vi "OP100 Indicators.vi"(8 "error in (no error)":errorcluster, 10 "Array":refnum<vi>[](array[refnum]), 11 "OUTPUT INDICATOR in":T1) -> (0 "error out":errorcluster, 3 "OUTPUT INDICATOR out":T1)   [LabVIEW 2017]
uses:
  2f4ed2d2-b3e5-497f-b08f-b9010f661fe3.vi
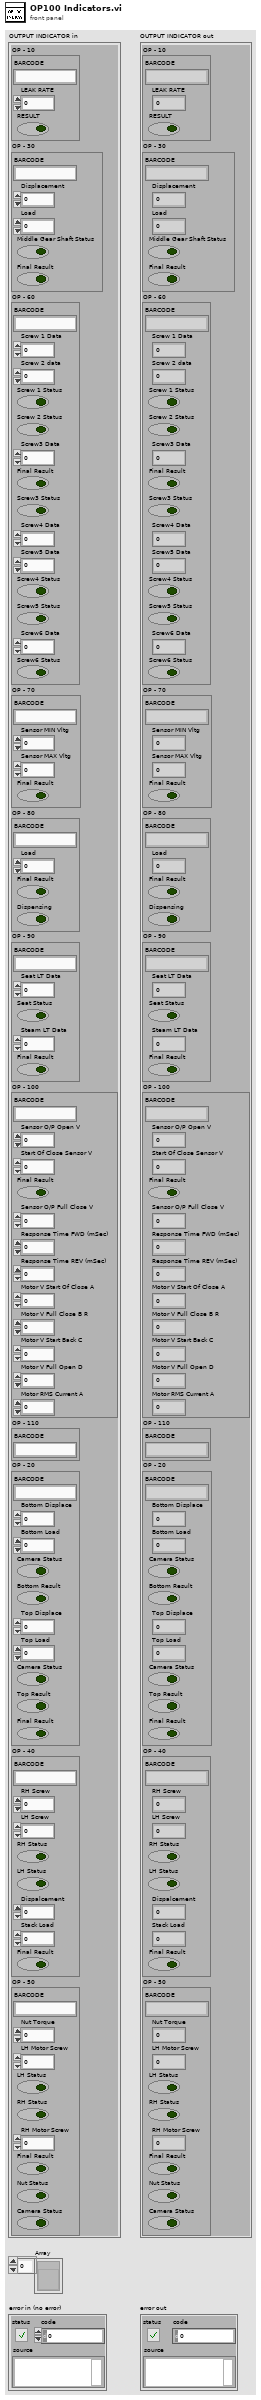
[diagram p1: front panel]
types:
  T1 = cluster{"OP - 10":cluster{"BARCODE":string, "LEAK RATE":dbl, "RESULT":bool}, "OP - 30":cluster{"BARCODE":string, "Displacement":dbl, "Load":dbl, "Middle Gear Shaft Status":bool, "Final Result":bool}, "OP - 60":cluster{"BARCODE":string, "Screw 1 Data":dbl, "Screw 2 data":dbl, "Screw 1 Status":bool, "Screw 2 Status":bool, "Screw3 Data":dbl, "Final Result":bool, "Screw3 Status":bool, "Screw4 Data":dbl, "Screw5 Data":dbl, "Screw4 Status":bool, "Screw5 Status":bool, "Screw6 Data":dbl, "Screw6 Status":bool}, "OP - 70":cluster{"BARCODE":string, "Sensor MIN Vltg":dbl, "Sensor MAX Vltg":dbl, "Final Result":bool}, "OP - 80":cluster{"BARCODE":string, "Load":dbl, "Final Result":bool, "Dispensing":bool}, "OP - 90":cluster{"BARCODE":string, "Seat LT Data":dbl, "Seat Status":bool, "Steam LT Data":dbl, "Final Result":bool}, "OP - 100":cluster{"BARCODE":string, "Sensor O/P Open V":dbl, "Start Of Close Sensor V":dbl, "Final Result":bool, "Sensor O/P Full Close V":dbl, "Response Time FWD (mSec)":dbl, "Response Time REV (mSec)":dbl, "Motor V Start Of Close A":dbl, "Motor V Full Close B R":dbl, "Motor V Start Back C":dbl, "Motor V Full Open D":dbl, "Motor RMS Current A":dbl}, "OP - 110":cluster{"BARCODE":string}, "OP - 20":cluster{"BARCODE":string, "Bottom Displace":dbl, "Bottom Load":dbl, "Camera Status":bool, "Bottom Result":bool, "Top Displace":dbl, "Top Load ":dbl, "Camera Status":bool, "Top Result":bool, "Final Result":bool}, "OP - 40":cluster{"BARCODE":string, "RH Screw":dbl, "LH Screw ":dbl, "RH Status":bool, "LH Status":bool, "Dispalcement ":dbl, "Stack Load ":dbl, "Final Result":bool}, "OP - 50":cluster{"BARCODE":string, "Nut Torque":dbl, "LH Motor Screw":dbl, "LH Status":bool, "RH Status":bool, "RH Motor Screw":dbl, "Final Result":bool, "Nut Status":bool, "Camera Status":bool}}
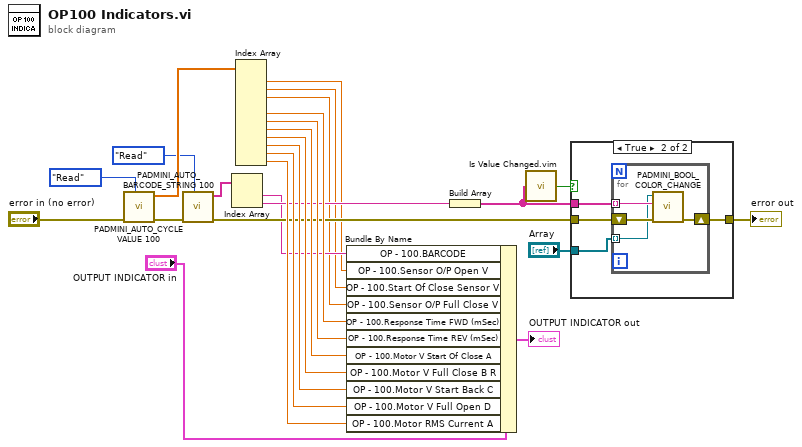
[diagram p0: block diagram]
diagram:
  n1 = call "PADMINI_AUTO_CYCLE VALUE 100.vi"("Enum"=enum16{"Read", "Write"}."Read", "error in (no error)"="error in (no error)") -> ("error out"=w11:errorcluster, "Input 2"=w14:sgl[])  [unwired: 8 in]
  n2 = call "PADMINI_AUTO_BARCODE_STRING 100.vi"("Enum"=enum16{"Read", "Write"}."Read", "error in (no error)"=w11) -> ("error out"=w12:errorcluster, "Input 2"=w17:string[])  [unwired: 8 in]
  n3 = Index Array(array=w17) -> (element #1=w4:string, element #2=w6:string)  [unwired: 2 in]
  n4 = Index Array(array=w14) -> (element #1=w3:sgl, element #2=w2:sgl, element #3=w1:sgl, element #5=w18:sgl, element #6=w19:sgl, element #7=w20:sgl, element #8=w21:sgl, element #9=w22:sgl, element #10=w23:sgl, element #11=w24:sgl)  [unwired: 11 in, 1 out]
  n5 = Bundle By Name(cluster="OUTPUT INDICATOR in", "OP - 100.BARCODE"=w4, "OP - 100.Sensor O/P Open V"=w3, "OP - 100.Start Of Close Sensor V"=w2, "OP - 100.Sensor O/P Full Close V"=w1, "OP - 100.Response Time FWD (mSec)"=w18, "OP - 100.Response Time REV (mSec)"=w19, "OP - 100.Motor V Start Of Close A"=w20, "OP - 100.Motor V Full Close B R"=w21, "OP - 100.Motor V Start Back C"=w22, "OP - 100.Motor V Full Open D"=w23, "OP - 100.Motor RMS Current A"=w24) -> (→"OUTPUT INDICATOR out":T1)
  n6 = Build Array(w6) -> (w7:string[])
  n7 = call "Is Value Changed.vim"("value"=w7) -> ("changed or first call?"=w5:bool)
  n8 = case shown="True" w5 {
    tunnel: [w26 w30] -> w13
    tunnel: w7 -> [_ w29]
    tunnel: w12 -> [w26 w28]
    tunnel: "Array" -> [_ w27]
    frame False {
    }
    frame True {
      n9 = for {
        tunnel: w29 -> [w33] mode=indexing
        shift-right: [w34] -> w30
        shift-left: w28 -> [w32]
        tunnel: w27 -> [w31] mode=indexing
        n10 = call "PADMINI_BOOL_COLOR_CHANGE.vi"("error in (no error)"=w32, "Input Result"=w33, "Boolean in"=w31) -> ("error out"=w34:errorcluster)  [unwired: 8 in]
      }
    }
  }
  "error out" <- w13
